vi "全局SQL.vi"() -> ()   [LabVIEW 2018]
panel:
  in  "udl":string="fed.udl"
  in  "table":string="CheckData"
  in  "cDefine48":string
  in  "cDefine47":string
  in  "cDefine46":string
  in  "cDefine45":string
  in  "cDefine44":string
  in  "cDefine43":string
  in  "cDefine42":string
  in  "cDefine41":string
  in  "cDefine40":string
  in  "cDefine39":string
  in  "cDefine38":string
  in  "cDefine37":string
  in  "cDefine31":string
  in  "cDefine32":string
  in  "cDefine33":string
  in  "cDefine34":string
  in  "cDefine35":string
  in  "cDefine36":string
  in  "cDefine30":string
  in  "cDefine29":string
  in  "cDefine28":string
  in  "cDefine27":string
  in  "cDefine26":string
  in  "cDefine25":string
  in  "cDefine24":string
  in  "cDefine23":string
  in  "cDefine22":string
  in  "cDefine21":string
  in  "cDefine20":string
  in  "cDefine19":string
  in  "Columns":string[](array[string])=["cMacCode", "cInvCode", "cCheckDate", "cCheckNo", "cState", "cDefine1", "cDefine2", "cDefine3", "cDefine4", "cDefine5", "cDefine6", "cDefine7", "cDefine8", "cDefine9", "cDefine10", "cDefine11", "cDefine12", "cDefine13", "cDefine14", "cDefine15", "cDefine16", "cDefine17", "cDefine18", "cDefine19", "cDefine20", "cDefine21", "cDefine22", "cDefine23", "cDefine24", "cDefine25", "cDefine26", "cDefine27", "cDefine28", "cDefine29", "cDefine30", "cDefine31", "cDefine32", "cDefine33", "cDefine34", "cDefine35", "cDefine36", "cDefine37", "cDefine38", "cDefine39", "cDefine40", "cDefine41", "cDefine42", "cDefine43", "cDefine44", "cDefine45", "cDefine46", "cDefine47", "cDefine48"]
  in  "cMacCode":string="1-C-000"
  in  "cInvCode":string
  in  "cCheckDate":string="2018-01-01 00:00:01"
  in  "cCheckNo":string="00000"
  in  "cState":string
  in  "cDefine1":string
  in  "cDefine2":string
  in  "cDefine3":string
  in  "cDefine4":string
  in  "cDefine5":string
  in  "cDefine6":string
  in  "cDefine7":string
  in  "cDefine8":string
  in  "cDefine9":string
  in  "cDefine10":string
  in  "cDefine11":string
  in  "cDefine12":string
  in  "cDefine13":string
  in  "cDefine14":string
  in  "cDefine15":string
  in  "cDefine16":string
  in  "cDefine17":string
  in  "cDefine18":string
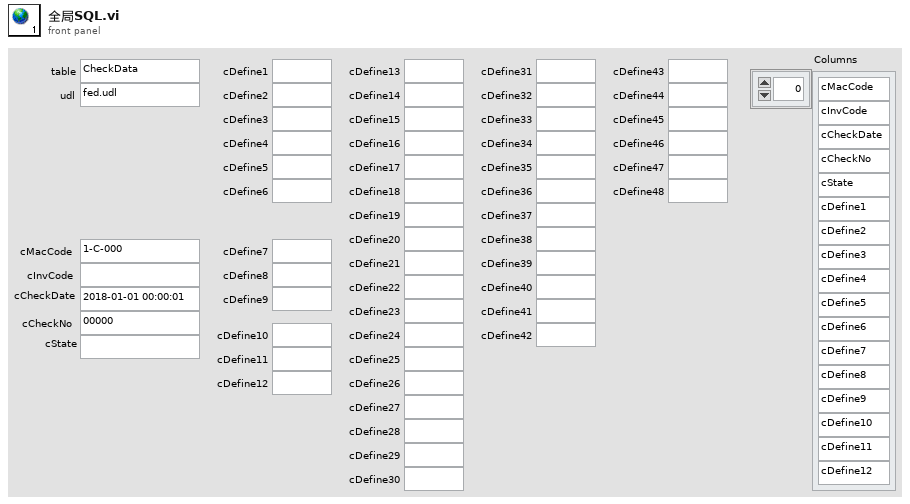
[diagram p1: front panel]
diagram:
